vi "Stack Control.vi"(6 "Feeder Mode Enabled":bool, 8 "Disable Stack":bool, 10 "Eject":bool, 11 "Suck":bool) -> (0 "frisbee counter":i16, 2 "Full Stack":bool, 3 "Empty Stack":bool, 5 "Is Sucking?":bool)   [LabVIEW 2012]
uses:
  BotStatus.vi
  Motors Values.vi
panel:
  # "Cannon"
  # "InFlipper"
  # "FlipperAtPlace"
  # "Middle"
  # "Bottom"
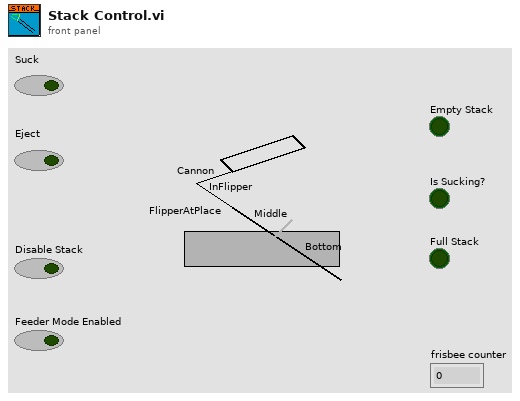
[diagram p1: front panel]
types:
  T1 = cluster{"Middle":bool, "InCannon":bool, "InFlipper":bool, "FlipperAtPlace":bool, "Bottom":bool, "FrisbeeDirection":bool}
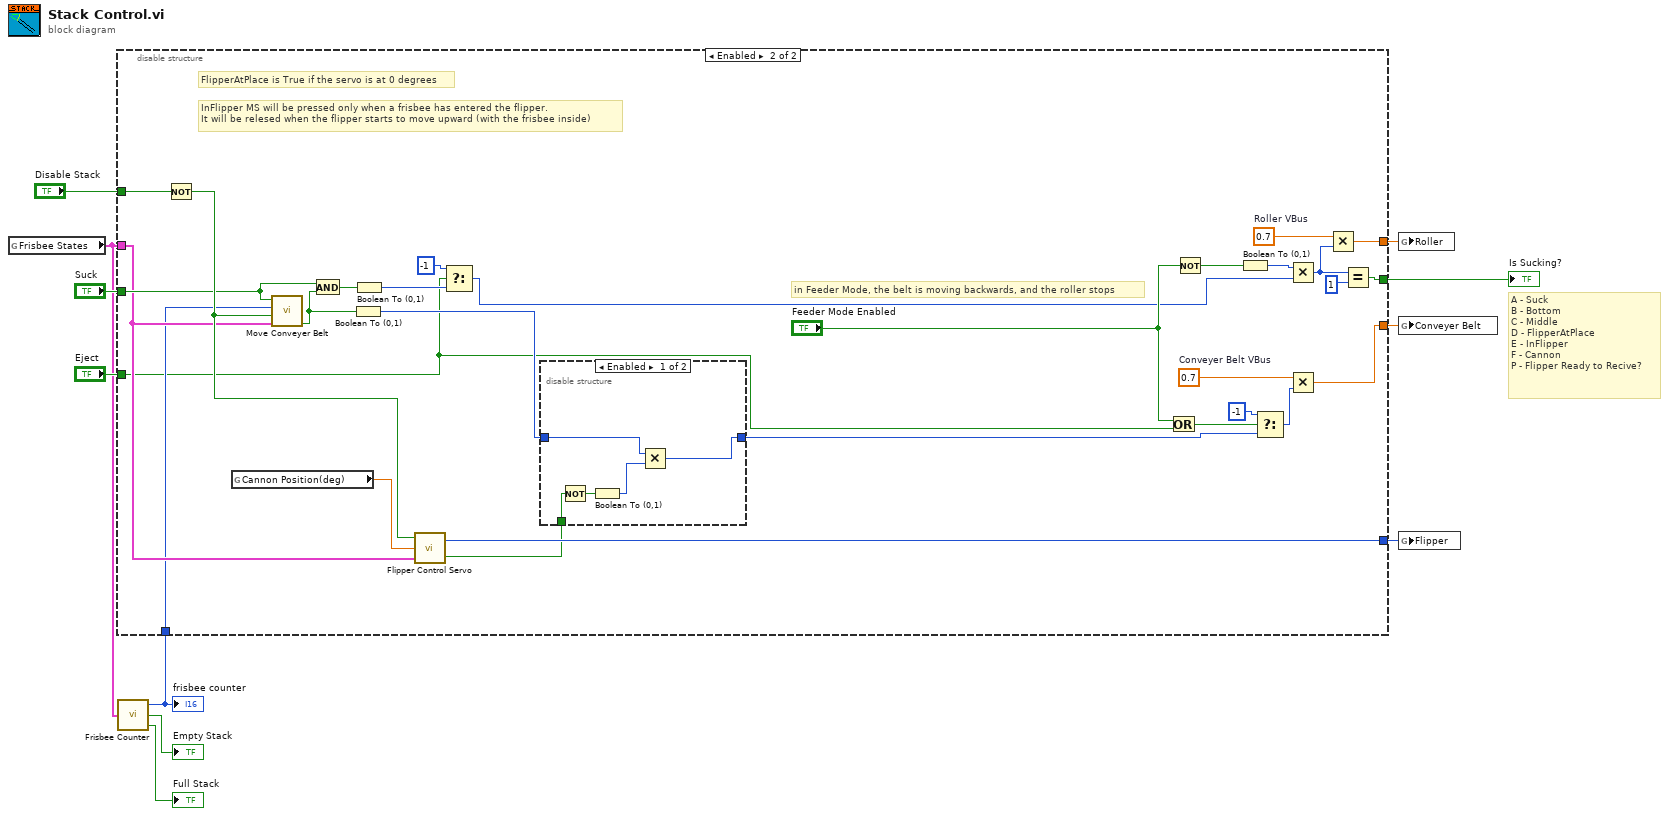
[diagram p0: block diagram]
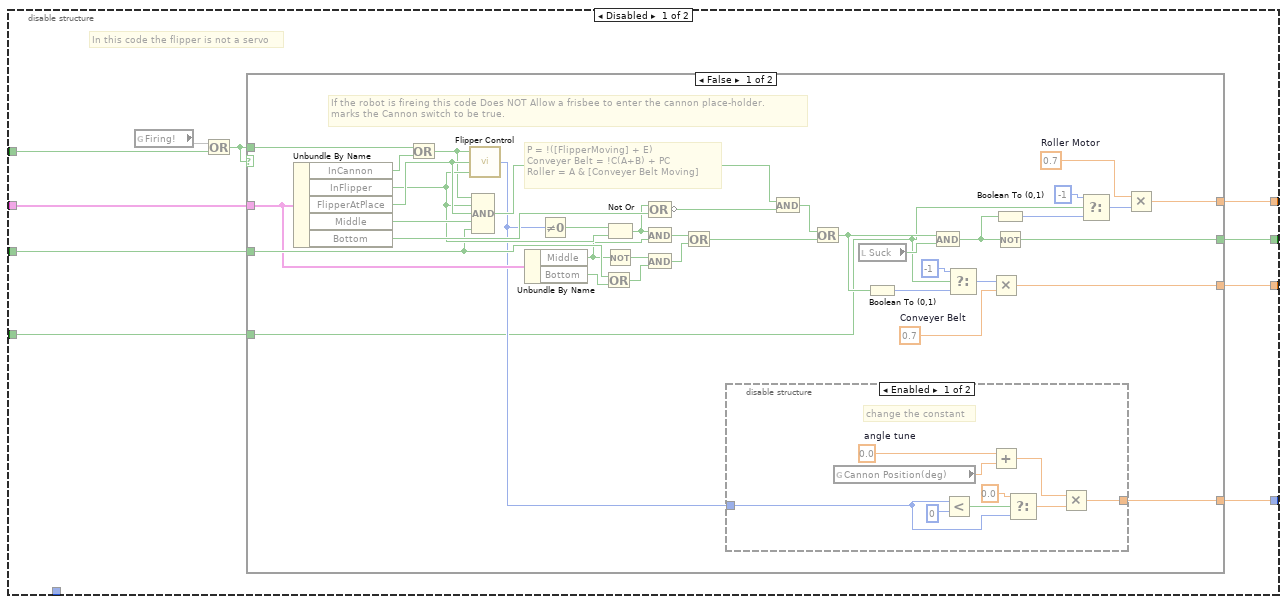
[diagram p2: hidden frame]
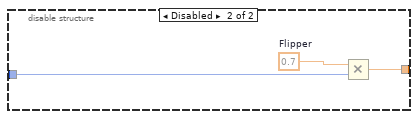
[diagram p3: hidden frame]
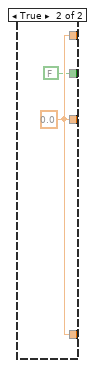
[diagram p4: hidden frame]
diagram:
  # "A - Suck\nB - Bottom\nC - Middle\nD - FlipperAtPlace\nE - InFlipper\nF - Cannon\nP - Flipper Ready to Recive?"
  n1 = global read "BotStatus.vi" "Frisbee States"() -> (w4:T1)
  n2 = call "Frisbee Counter.vi"("Frisbee States"=w4) -> ("frisbee counter"=w1:i16, "Stack Empty?"=→"Empty Stack":bool, "Stack Full?"=→"Full Stack":bool)
  "frisbee counter" <- w1
  n3 = disable-structure shown="Enabled" {
    disable-tunnel: "Suck" -> [w21 w77]
    disable-tunnel: [w20 w97] -> w10
    disable-tunnel: [w19 w98] -> w9
    disable-tunnel: w4 -> [w18 w76]
    disable-tunnel: "Disable Stack" -> [w15 w99]
    disable-tunnel: "Eject" -> [w14 w74]
    disable-tunnel: [w13 w92] -> w6
    disable-tunnel: [w12 w91] -> w5
    disable-tunnel: w1 -> [_ w75]
    frame Disabled {
      # "In this code the flipper is not a servo"
      n4 = global read "BotStatus.vi" "Firing!"() -> (w17)
      n5 = Or(x=w17, y=w15) -> (x .or. y?=w16:bool)
      n6 = case shown="False" w16 {
        tunnel: w21 -> [w48 _]
        tunnel: [w29 w73] -> w20
        tunnel: w16 -> [w28 _]
        tunnel: [w27 w73] -> w19
        tunnel: [w24 w73] -> w13
        tunnel: w18 -> [w26 _]
        tunnel: w14 -> [w23 _]
        tunnel: [w22 FALSE] -> w12
        frame False {
          w40 = 0.7  # Conveyer Belt
          w39 = 0.7  # Roller Motor
          # "If the robot is fireing this code Does NOT Allow a frisbee to enter the cannon place-holder.\nmarks the Cannon switch to be true."
          # "P = !([FlipperMoving] + E)\nConveyer Belt = !C(A+B) + PC\nRoller = A & [Conveyer Belt Moving]"
          n7 = Unbundle By Name(w26) -> ("InCannon"=w31:bool, "InFlipper"=w55:bool, "FlipperAtPlace"=w59:bool, "Middle"=w58:bool, "Bottom"=w57:bool)
          n8 = Or(x=w28, y=w31) -> (x .or. y?=w30:bool)
          n9 = call "Flipper Control.vi"("InFlipper"=w55, "FlipperAtPlace"=w59, "FrisbiInCannon"=w30) -> ("Flipper Direction"=w25:i32)
          n10 = Compound Arithmetic op=AND(w30, w55, w59, w58, w48) -> (w54:bool)
          n11 = Unbundle By Name(w26) -> ("Middle"=w41:bool, "Bottom"=w49:bool)
          n12 = Not Equal To 0?(x=w25) -> (x != 0?=w56:bool)
          n13 = Or(x=w48, y=w49) -> (x .or. y?=w47:bool)
          n14 = Not Or(1:w55, 2:w56) -> (0:w38:bool)
          n15 = Not(x=w41) -> (.not. x?=w46:bool)
          n16 = And(x=w38, y=w41) -> (x .and. y?=w51:bool)
          n17 = And(x=w46, y=w47) -> (x .and. y?=w45:bool)
          n18 = Compound Arithmetic op=OR(w38, w57) -> (invert w53:bool)
          n19 = Or(x=w51, y=w45) -> (x .or. y?=w50:bool)
          n20 = disable-structure shown="Enabled" {
            disable-tunnel: w25 -> [w61 w70]
            disable-tunnel: [w67 w71] -> w24
            frame Enabled {
              w65 = 0.0  # angle tune
              # "change the constant"
              n21 = global read "BotStatus.vi" "Cannon Position(deg)"() -> (w66:dbl)
              n22 = Less?(x=w61, y=i16 0) -> (x < y?=w63:bool)
              n23 = Add(x=w65, y=w66) -> (x+y=w68:dbl)
              n24 = Select(t=0.0, s=w63, f=w61) -> (s? t:f=w60:dbl)
              n25 = Multiply(x=w68, y=w60) -> (x*y=w67:dbl)
            }
            frame Disabled {
              w69 = 0.7  # Flipper
              n26 = Multiply(x=w69, y=w70) -> (x*y=w71:dbl)
            }
          }
          n27 = And(x=w54, y=w53) -> (x .and. y?=w52:bool)
          n28 = Or(x=w52, y=w50) -> (x .or. y?=w43:bool)
          n29 = local read "Suck"() -> (w42:bool)
          n30 = Boolean To (0,1)(Boolean=w43) -> (0, 1=w37:i16)
          n31 = And(x=w43, y=w42) -> (x .and. y?=w44:bool)
          n32 = Select(t=i16 -1, s=w23, f=w37) -> (s? t:f=w36:i16)
          n33 = Multiply(x=w36, y=w40) -> (x*y=w27:dbl)
          n34 = Boolean To (0,1)(Boolean=w44) -> (0, 1=w34:i16)
          n35 = Not(x=w44) -> (.not. x?=w22:bool)
          n36 = Select(t=i16 -1, s=w23, f=w34) -> (s? t:f=w33:i16)
          n37 = Multiply(x=w39, y=w33) -> (x*y=w29:dbl)
        }
        frame True {
          w73 = 0.0
        }
      }
    }
    frame Enabled {
      w101 = 0.7  # Roller VBus
      w102 = 0.7  # Conveyer Belt VBus
      # "in Feeder Mode, the belt is moving backwards, and the roller stops"
      # "FlipperAtPlace is True if the servo is at 0 degrees"
      # "InFlipper MS will be pressed only when a frisbee has entered the flipper.\nIt will be relesed when the flipper starts to move upward (with the frisbee inside)"
      n38 = Not(x=w99) -> (.not. x?=w84:bool)
      n39 = global read "BotStatus.vi" "Cannon Position(deg)"() -> (w85:dbl)
      n40 = call "Move Conveyer Belt.vi"("Frisbee States"=w76, "Enable Stack"=w84, "frisbee counter"=w75, "Suck"=w77) -> ("move conveyer belt"=w81:bool)  [unwired: 5 in]
      n41 = And(x=w77, y=w81) -> (x .and. y?=w100:bool)
      n42 = Boolean To (0,1)(Boolean=w81) -> (0, 1=w79:i16)
      n43 = Boolean To (0,1)(Boolean=w100) -> (0, 1=w93:i16)
      n44 = call "Flipper Control Servo.vi"("Frisbee States"=w76, "Cannon Position(deg)"=w85, "Enable Stack"=w84) -> ("Stop Conveyer Belt"=w82:bool, "Set Flipper's Servos Angle"=w92:i32)
      n45 = Select(t=i16 -1, s=w74, f=w93) -> (s? t:f=w80:i16)
      n46 = disable-structure shown="Enabled" {
        disable-tunnel: [w103 w108] -> w78
        disable-tunnel: w79 -> [w105 w108]
        disable-tunnel: w82 -> [w107 _]
        frame Enabled {
          n47 = Not(x=w107) -> (.not. x?=w106:bool)
          n48 = Boolean To (0,1)(Boolean=w106) -> (0, 1=w104:i16)
          n49 = Multiply(x=w105, y=w104) -> (x*y=w103:i16)
        }
        frame Disabled {
        }
      }
      n50 = Or(x="Feeder Mode Enabled", y=w74) -> (x .or. y?=w89:bool)
      n51 = Not(x="Feeder Mode Enabled") -> (.not. x?=w87:bool)
      n52 = Boolean To (0,1)(Boolean=w87) -> (0, 1=w86:i16)
      n53 = Select(t=i16 -1, s=w89, f=w78) -> (s? t:f=w95:i16)
      n54 = Multiply(x=w86, y=w80) -> (x*y=w83:i16)
      n55 = Multiply(x=w102, y=w95) -> (x*y=w98:dbl)
      n56 = Multiply(x=w101, y=w83) -> (x*y=w97:dbl)
      n57 = Equal?(x=w83, y=1) -> (x = y?=w91:bool)
    }
  }
  "Is Sucking?" <- w5
  n58 = global write "Motors Values.vi" "Roller"(w10) -> ()
  n59 = global write "Motors Values.vi" "Conveyer Belt"(w9) -> ()
  n60 = global write "Motors Values.vi" "Flipper"(w6) -> ()
